vi "convert para.vi"() -> ()   [LabVIEW 2010]
panel:
  in  "Choose Cycle Time (1: Fixed Time) 2":u16(ring)=1 items=["Variable Burst", "Fixed Time"]
  in  "Function (1: Heat) 2":u16(ring)=1 items=["Off", "Heat", "Cool"]
  in  "Process Output Type (0: 4 to 20 mA) 2":u16(ring) items=["4 to 20 mA", "0 to 20 mA", "0 to 5 V", "1 to 5 V", "0 to 10 V"]
  in  "Process Output Type (0: 4 to 20 mA)":u16(ring) items=["4 to 20 mA", "0 to 20 mA", "0 to 5 V", "1 to 5 V", "0 to 10 V"]
  in  "Function (1: Heat)":u16(ring)=1 items=["Off", "Heat", "Cool"]
  in  "Choose Cycle Time (1: Fixed Time)":u16(ring)=1 items=["Variable Burst", "Fixed Time"]
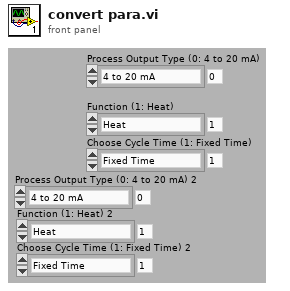
[diagram p1: front panel]
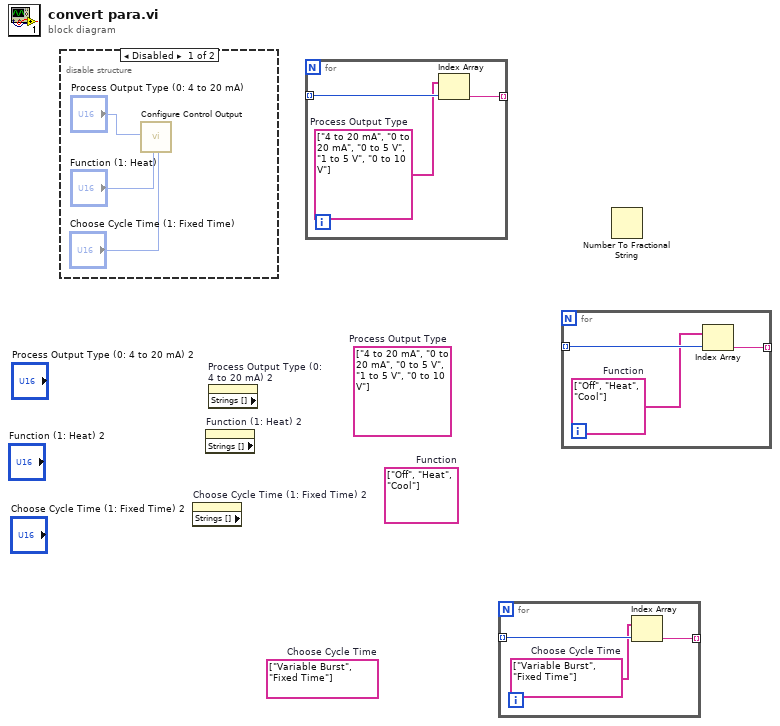
[diagram p0: block diagram]
diagram:
  (unwired) string[] ["Variable Burst", "Fixed Time"]  # Choose Cycle Time
  (unwired) string[] ["Off", "Heat", "Cool"]  # Function
  (unwired) string[] ["4 to 20 mA", "0 to 20 mA", "0 to 5 V", "1 to 5 V", "0 to 10 V"]  # Process Output Type
  n1 = disable-structure shown="Disabled" {
    frame Disabled {
      n2 = call "Configure Control Output.vi"("Process Output Type (0: 4 to 20 mA)"="Process Output Type (0: 4 to 20 mA)", "Function (1: Heat)"="Function (1: Heat)", "Choose Cycle Time (1: Fixed Time)"="Choose Cycle Time (1: Fixed Time)") -> ()  [unwired: 15 in, 2 out]
    }
    frame Enabled {
    }
  }
  n3 = property on="Choose Cycle Time (1: Fixed Time) 2" class="Ring (strict)" props=["Strings []"]() -> ()  [unwired: 2 in, 3 out]
  n4 = property on="Function (1: Heat) 2" class="Ring (strict)" props=["Strings []"]() -> ()  [unwired: 2 in, 3 out]
  n5 = property on="Process Output Type (0: 4 to 20 mA) 2" class="Ring (strict)" props=["Strings []"]() -> ()  [unwired: 2 in, 3 out]
  n6 = for {
    tunnel: _ -> [w6] mode=indexing
    tunnel: [w5] -> _ mode=indexing
    w4 = string[] ["4 to 20 mA", "0 to 20 mA", "0 to 5 V", "1 to 5 V", "0 to 10 V"]  # Process Output Type
    n7 = Index Array(array=w4, index=w6) -> (element=w5:string)
  }
  n8 = for {
    tunnel: _ -> [w9] mode=indexing
    tunnel: [w8] -> _ mode=indexing
    w7 = string[] ["Variable Burst", "Fixed Time"]  # Choose Cycle Time
    n9 = Index Array(array=w7, index=w9) -> (element=w8:string)
  }
  n10 = for {
    tunnel: _ -> [w12] mode=indexing
    tunnel: [w11] -> _ mode=indexing
    w10 = string[] ["Off", "Heat", "Cool"]  # Function
    n11 = Index Array(array=w10, index=w12) -> (element=w11:string)
  }
  n12 = Number To Fractional String() -> ()  [unwired: 4 in, 1 out]
